vi "ProximitySensor(SubVI).vi"(11 "prox_din":dbl) -> (1 "prox_out_range":bool, 2 "prox_max":dbl, 3 "prox":dbl, 4 "prox_min":dbl)   [LabVIEW 2017]
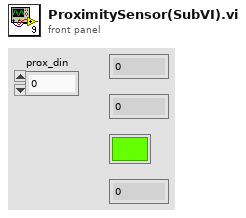
[diagram p1: front panel]
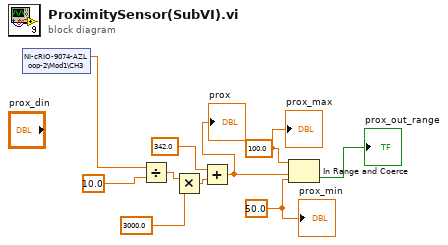
[diagram p0: block diagram]
diagram:
  w10 = 50.0 ("upper limit")
  w8 = 100.0 ("upper limit")
  n1 = shared-variable "NI-cRIO-9074-AZLoop-2\\Mod1\\CH3"() -> (w1:dbl)  [unwired: 1 in, 1 out]
  n2 = Divide(x=w1, y=10.0) -> (x/y=w3:dbl)
  n3 = Multiply(x=w3, y=3000.0) -> (x*y=w5:dbl)
  n4 = Add(x=342.0, y=w5) -> (x+y=w7:dbl)
  "prox" <- w7
  n5 = In Range and Coerce(upper limit=w8, x=w7, lower limit=w10) -> (In Range?=→"prox_out_range":bool)  [unwired: 1 out]
  "prox_min" <- w10
  "prox_max" <- w8
